vi "templates List Templates.vi"(8 "error in (no error)":errorcluster, 11 "Connection Refnum In\n(0,0: Open New)":T1) -> (0 "error out":errorcluster, 1 "Template Keys":T2, 3 "Connection Refnum In\n(0,0: Open New)":T1)   [LabVIEW 2011]
uses:
  Addons/internet/utils/keyedarr.llb/Keyed Array.ctl
  SI.LIB/ODBC/SQL Controls/Connection Refnum.ctl
  Addons/internet/utils/strutil.llb/Case Matching.ctl
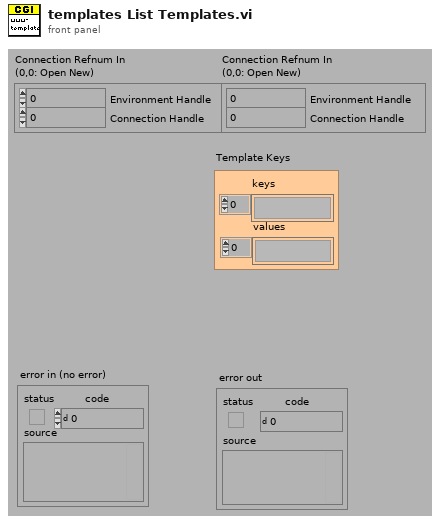
[diagram p1: front panel]
types:
  T1 = typedef "Connection Refnum.ctl" = cluster{"Environment Handle":i32, "Connection Handle":i32}
  T2 = typedef "Keyed Array.ctl" = cluster{"keys":string[], "values":string[]}
  T3 = typedef "Template Record.ctl" = cluster{"ixTemplate":i32, "sxTemplateId":string, "sDescription":string, "sCreator":string, "tCreationDate":timestamp, "sModifier":string, "tModifiedDate":timestamp, "sType":string, "sStyle":string, "sFormat":string, "dWidth":dbl, "dHeight":dbl, "sFilename":string, "sScript":string, "sLayout":string, "sEditor":string, "sStyleProcess":string}
  T4 = typedef "Case Matching.ctl" = enum16{"a != A", "a == A", "system"}
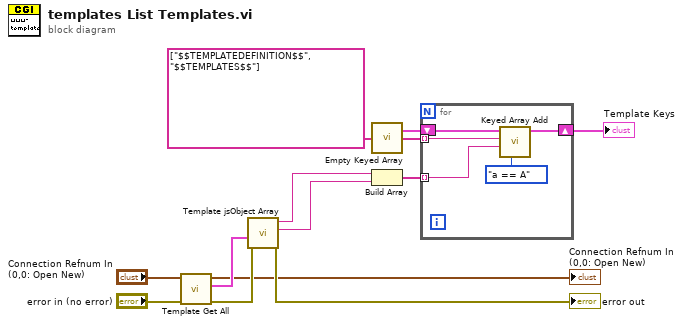
[diagram p0: block diagram]
diagram:
  n1 = call "Template Get All.vi"("error in (no error)"="error in (no error)", "Connection Refnum"="Connection Refnum In\n(0,0: Open New)") -> ("error out"=w2:errorcluster, "Templates"=w3:T3[], "Connection Refnum"=→"Connection Refnum In\n(0,0: Open New)":T1)  [unwired: 1 in, 6 out]
  n2 = call "Template jsObject Array.vi"("error in (no error)"=w2, "TEMPLATES (none)"=w3) -> ("error out"=→"error out":errorcluster, "Templates jsObject Array"=w4:string, "Template jsObject Definition"=w5:string)  [unwired: 2 in, 5 out]
  n3 = call "Empty Keyed Array.vi"() -> ("empty keyed array"=w12:T2)  [unwired: 3 out]
  n4 = Build Array(w5, w4) -> (w11:string[])
  n5 = for {
    shift-right: [w14] -> w10
    shift-left: w12 -> [w16]
    tunnel: string[] ["$$TEMPLATEDEFINITION$$", "$$TEMPLATES$$"] -> [w15] mode=indexing
    tunnel: w11 -> [w13] mode=indexing
    n6 = call "Keyed Array Add.vi"("case matching (sensitive)"=Case_Matching."a == A", "value"=w13, "key"=w15, "array in"=w16) -> ("array out"=w14:T2)  [unwired: 3 out]
  }
  "Template Keys" <- w10
